vi "215.Home (SubVI).vi"(8 "error in (no error)":errorcluster, 11 "VISA resource name":refnum<visa-resource-name>="COM7") -> (0 "error out":errorcluster, 1 "String":string, 2 "Connected":bool, 3 "VISA Out":refnum<visa-resource-name>)   [LabVIEW 2020]
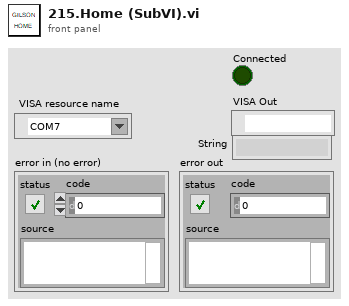
[diagram p1: front panel]
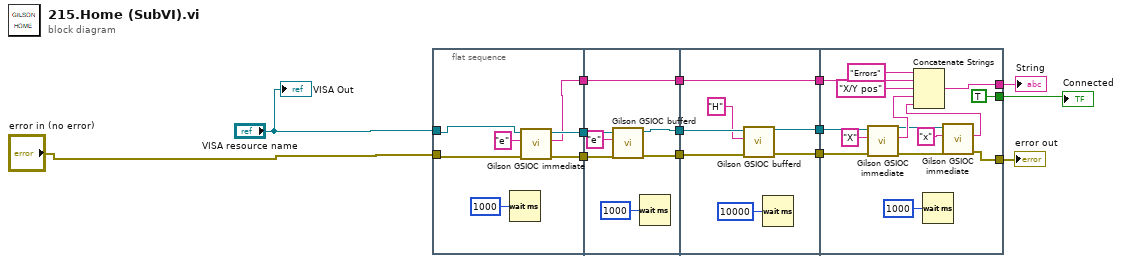
[diagram p0: block diagram]
diagram:
  n1 = flat-sequence {
    tunnel: "VISA resource name" -> [w19]
    tunnel: "error in (no error)" -> [w21]
    tunnel: [w18] -> w12
    tunnel: [w17] -> w11
    tunnel: [w15] -> w9
    tunnel: [w25] -> w14
    tunnel: [w24] -> w13
    tunnel: w12 -> [w28]
    tunnel: w11 -> [w26]
    tunnel: w9 -> [w22]
    tunnel: [w22] -> w7
    tunnel: w14 -> [w35]
    tunnel: w13 -> [w34]
    tunnel: [w31] -> w8
    tunnel: w7 -> [w31]
    tunnel: [w30] -> w6
    tunnel: [w29] -> w5
    tunnel: [TRUE ("Connected")] -> w10
    tunnel: w8 -> [w49]
    tunnel: w6 -> [w46]
    tunnel: w5 -> [w45]
    tunnel: [w41] -> w4
    tunnel: [w40] -> w3
    frame #0 {
      n2 = Wait (ms)(milliseconds to wait=u32 1000) -> ()  [unwired: 1 out]
      n3 = call <instrlib>:"Gilson GSIOC immediate.vi"("error in (no error)"=w21, "Immediate command"="e", "VISA resource name"=w19) -> ("error out"=w17:errorcluster, "Receive string"=w15:string, "VISA resource name"=w18:refnum<visa-resource-name>)  [unwired: 6 in]
    }
    frame #1 {
      n4 = call <instrlib>:"Gilson GSIOC bufferd.vi"("error in (no error)"=w26, "Bufferd command"="e", "VISA resource name"=w28) -> ("error out"=w25:errorcluster, "VISA resource name out"=w24:refnum<visa-resource-name>)  [unwired: 6 in, 1 out]
      n5 = Wait (ms)(milliseconds to wait=u32 1000) -> ()  [unwired: 1 out]
    }
    frame #2 {
      n6 = call <instrlib>:"Gilson GSIOC bufferd.vi"("error in (no error)"=w35, "Bufferd command"="H", "VISA resource name"=w34) -> ("error out"=w30:errorcluster, "VISA resource name out"=w29:refnum<visa-resource-name>)  [unwired: 6 in, 1 out]
      n7 = Wait (ms)(milliseconds to wait=u32 10000) -> ()  [unwired: 1 out]
    }
    frame #3 {
      n8 = call <instrlib>:"Gilson GSIOC immediate.vi"("error in (no error)"=w46, "Immediate command"="X", "VISA resource name"=w45) -> ("error out"=w42:errorcluster, "Receive string"=w43:string, "VISA resource name"=w38:refnum<visa-resource-name>)  [unwired: 6 in]
      n9 = Wait (ms)(milliseconds to wait=u32 1000) -> ()  [unwired: 1 out]
      n10 = call <instrlib>:"Gilson GSIOC immediate.vi"("error in (no error)"=w42, "Immediate command"="x", "VISA resource name"=w38) -> ("error out"=w41:errorcluster, "Receive string"=w37:string)  [unwired: 6 in, 1 out]
      n11 = Concatenate Strings("Errors" ("string"), w49, "X/Y pos" ("string"), w43, w37) -> (w40:string)
    }
  }
  "VISA Out" <- "VISA resource name"
  "error out" <- w4
  "Connected" <- w10
  "String" <- w3
